vi "ConfigParams - Set - UDPData.vi"(7 "UDP Data Enable":bool=TRUE, 8 "error in (no error)":errorcluster, 9 "UDPDataPeriod_mS":u32=5, 10 "UDP Data Port":u16=54321, 11 "Ethernet in":refnum<class "ENET_BS1201.lvclass">) -> (0 "error out":errorcluster, 3 "Ethernet out":refnum<class "ENET_BS1201.lvclass">)   [LabVIEW 2021, in "BS120x Driver.lvlib" / "ENET_BS1201.lvclass"]
uses:
  ENET_BS1201.lvclass
panel:
  # "[UDPData]\nUDPDataEnable = True\nUDPDataPort = 54322\nUDPDataPeriod_mS = 5"
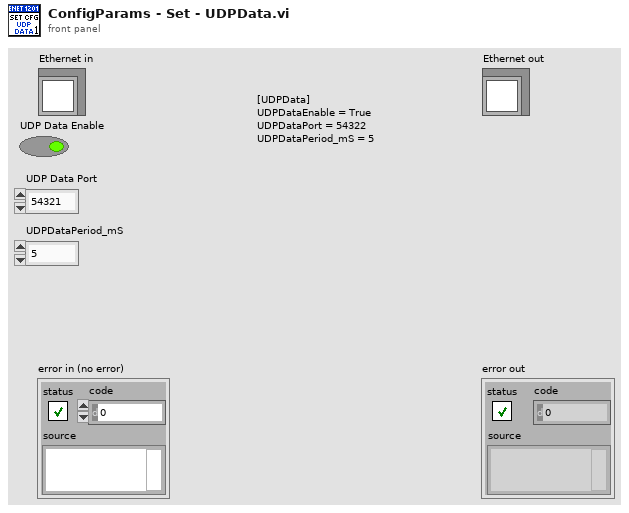
[diagram p1: front panel]
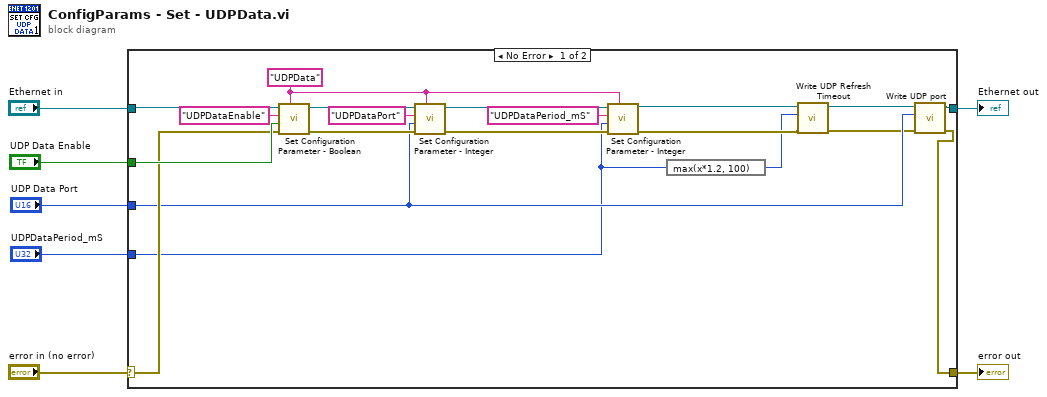
[diagram p0: block diagram]
diagram:
  n1 = case shown="No Error" "error in (no error)" {
    selector: "error in (no error)" -> [w18 w29]
    tunnel: [w9 w29] -> w6
    tunnel: [w16 w28] -> w4
    tunnel: "Ethernet in" -> [w27 w28]
    tunnel: "UDP Data Enable" -> [w25 _]
    tunnel: "UDP Data Port" -> [w15 _]
    tunnel: "UDPDataPeriod_mS" -> [w14 _]
    frame No Error {
      w20 = "UDPData" ("Section")
      n2 = call-dynamic "Set Configuration Parameter - Boolean.vi"("Section"=w20, "error in (no error)"=w18, "Value"=w25, "Key"="UDPDataEnable", "Ethernet in"=w27) -> ("error out"=w17:errorcluster, "Ethernet out"=w24:refnum<class "ENET_BS1201.lvclass">)  [unwired: 5 in]
      n3 = call-dynamic "Set Configuration Parameter - Integer.vi"("Section"=w20, "error in (no error)"=w17, "Value"=w15, "Key"="UDPDataPort", "Ethernet in"=w24) -> ("error out"=w21:errorcluster, "Ethernet out"=w22:refnum<class "ENET_BS1201.lvclass">)  [unwired: 5 in]
      n4 = call-dynamic "Set Configuration Parameter - Integer.vi"("Section"=w20, "error in (no error)"=w21, "Value"=w14, "Key"="UDPDataPeriod_mS", "Ethernet in"=w22) -> ("error out"=w10:errorcluster, "Ethernet out"=w13:refnum<class "ENET_BS1201.lvclass">)  [unwired: 5 in]
      n5 = expression code="max(x*1.2, 100)"(w14) -> (w8:u32)
      n6 = call-dynamic "Write UDP Refresh Timeout.vi"("error in (no error)"=w10, "UDP Refresh Timeout"=w8, "ENET_BS120x in"=w13) -> ("error out"=w11:errorcluster, "ENET_BS120x out"=w12:refnum<class "ENET_BS1201.lvclass">)  [unwired: 7 in]
      n7 = call-dynamic "Write UDP port.vi"("error in (no error)"=w11, "UDP port"=w15, "ENET_BS120x in"=w12) -> ("error out"=w9:errorcluster, "ENET_BS120x out"=w16:refnum<class "ENET_BS1201.lvclass">)  [unwired: 7 in]
    }
    frame Error {
    }
  }
  "error out" <- w6
  "Ethernet out" <- w4
